vi "Test Keithley 24xx.vi"() -> ()   [LabVIEW 2020, in "Keithley 24xx.lvclass"]
uses:
  Keithley 24xx.lvclass
  C:/Sandbox/Git_Sandbox/WiSpry Test Framework source code (LV20)/WiSpry Test Framework/Instruments/Instrument.lvclass
  Instrument.lvclass/Instrument.ctl
  Instrument.lvclass
panel:
  out "Current":dbl
  out "Voltage":dbl
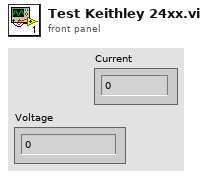
[diagram p1: front panel]
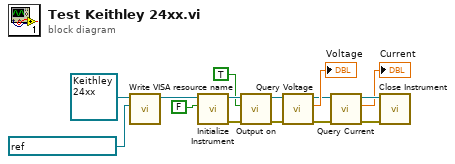
[diagram p0: block diagram]
diagram:
  n1 = call "Write VISA resource name.vi"("VISA resource name"=refnum<visa-resource-name> "GPIB0::2::INSTR", "Instrument in"=refnum<class "Keithley 24xx.lvclass"> refnum ("Keithley 24xx.lvclass")) -> ("Instrument out"=w15:refnum<class "Keithley 24xx.lvclass">)  [unwired: 9 in]
  n2 = call-dynamic "Initialize Instrument.vi"("Reset"=FALSE, "Keithley 24xx in"=w15) -> ("error out"=w8:errorcluster, "Keithley 24xx out"=w9:refnum<class "Keithley 24xx.lvclass">)  [unwired: 8 in]
  n3 = call-dynamic "Output on.vi"("error in (no error)"=w8, "Output On"=TRUE, "Keithley 24xx in"=w9) -> ("error out"=w7:errorcluster, "Keithley 24xx out"=w10:refnum<class "Keithley 24xx.lvclass">)  [unwired: 7 in]
  n4 = call-dynamic "Query Voltage.vi"("error in (no error)"=w7, "Keithley 24xx in"=w10) -> ("error out"=w5:errorcluster, "Voltage"=→"Voltage":dbl, "Keithley 24xx out"=w4:refnum<class "Keithley 24xx.lvclass">)  [unwired: 7 in]
  n5 = call-dynamic "Query Current.vi"("error in (no error)"=w5, "Keithley 24xx in"=w4) -> ("error out"=w3:errorcluster, "Current"=→"Current":dbl, "Keithley 24xx out"=w2:refnum<class "Keithley 24xx.lvclass">)  [unwired: 7 in]
  n6 = call-dynamic "Close Instrument.vi"("error in (no error)"=w3, "Instrument in"=w2) -> ()  [unwired: 8 in, 2 out]
